vi "IO_Switch_#2(S2).vi"(8 "error in":errorcluster, 10 "Output":T1(ring)=enum."AVR (J3)", 11 "Input":T2(ring)=enum."Splitter") -> (0 "error out":errorcluster, 2 "Verfied":bool, 3 "Switches":string)   [LabVIEW 2012]
panel:
  # "IO Switch #2 (S2)"
  # "Switch Output"
  # "Switch Input"
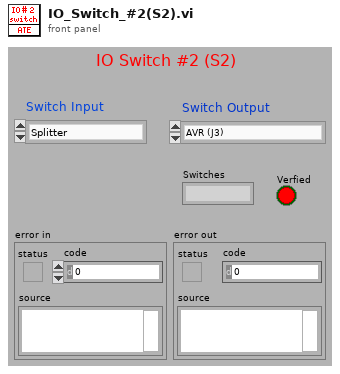
[diagram p1: front panel]
types:
  T1 = enum16{"NONE", "AVR (J3)", "Signal Out Switch (S3)", "Power Meter Switch (S5)", "Reversing Switch", "2W Term (TM1)"}
  T2 = enum16{"NONE", "AVR (J3)", "Splitter", "Signal Out Switch (S3)", " 2W Term (TM1)", "Reversing Switch", "Power Meter Switch"}
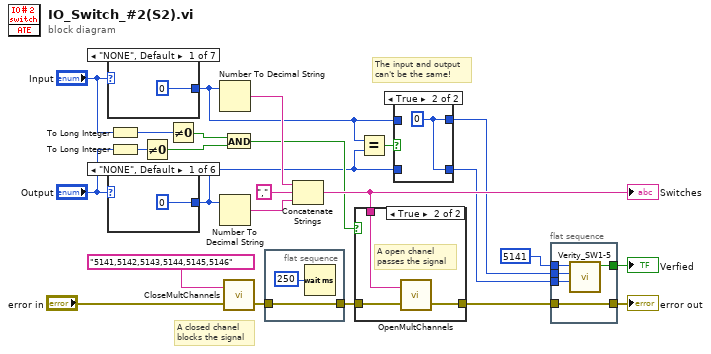
[diagram p0: block diagram]
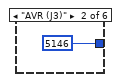
[diagram p3: hidden frame]
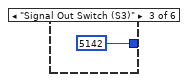
[diagram p4: hidden frame]
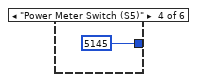
[diagram p5: hidden frame]
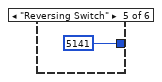
[diagram p6: hidden frame]
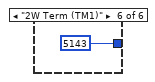
[diagram p7: hidden frame]
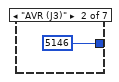
[diagram p8: hidden frame]
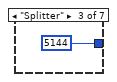
[diagram p9: hidden frame]
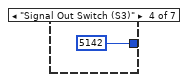
[diagram p10: hidden frame]
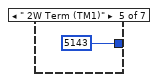
[diagram p11: hidden frame]
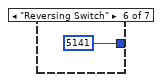
[diagram p12: hidden frame]
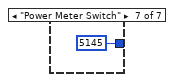
[diagram p13: hidden frame]
diagram:
  # "The input and output\ncan't be the same!"
  # "A closed chanel\nblocks the signal"
  n1 = case shown="\"NONE\", Default" "Input" {
    tunnel: [0 ("Switch ID") 5146 ("Switch ID") 5144 ("Switch ID") 5142 ("Switch ID") 5143 ("Switch ID") 5141 ("Switch ID") 5145 ("Switch ID")] -> w7
    frame "NONE", Default {
    }
    frame "AVR (J3)" {
    }
    frame "Splitter" {
    }
    frame "Signal Out Switch (S3)" {
    }
    frame " 2W Term (TM1)" {
    }
    frame "Reversing Switch" {
    }
    frame "Power Meter Switch" {
    }
  }
  n2 = case shown="\"NONE\", Default" "Output" {
    tunnel: [0 ("Switch ID") 5146 ("Switch ID") 5142 ("Switch ID") 5145 ("Switch ID") 5141 ("Switch ID") 5143 ("Switch ID")] -> w8
    frame "NONE", Default {
    }
    frame "AVR (J3)" {
    }
    frame "Signal Out Switch (S3)" {
    }
    frame "Power Meter Switch (S5)" {
    }
    frame "Reversing Switch" {
    }
    frame "2W Term (TM1)" {
    }
  }
  n3 = To Long Integer(number="Input") -> (32bit integer=w14:i32)
  n4 = To Long Integer(number="Output") -> (32bit integer=w13:i32)
  n5 = Not Equal To 0?(x=w13) -> (x != 0?=w12:bool)
  n6 = Not Equal To 0?(x=w14) -> (x != 0?=w11:bool)
  n7 = Number To Decimal String(number=w7) -> (decimal integer string=w17:string)  [unwired: 1 in]
  n8 = Number To Decimal String(number=w8) -> (decimal integer string=w18:string)  [unwired: 1 in]
  n9 = And(x=w11, y=w12) -> (x .and. y?=w10:bool)
  n10 = call "CloseMultChannels.vi"("error in (no error)"="error in", "Channels to be closed"="5141,5142,5143,5144,5145,5146" ("Channels to be opened")) -> ("error out"=w20:errorcluster)  [unwired: 1 in]
  n11 = flat-sequence {
    tunnel: w20 -> [w38]
    tunnel: [w38] -> w19
    frame #0 {
      n12 = Wait (ms)(milliseconds to wait=u32 250) -> ()  [unwired: 1 out]
    }
  }
  n13 = Concatenate Strings(w17, ",", w18) -> (w21:string)
  "Switches" <- w21
  n14 = case shown="True" w10 {
    tunnel: w19 -> [w40 w42]
    tunnel: w21 -> [_ w43]
    tunnel: [w40 w41] -> w2
    frame False {
    }
    frame True {
      # "A open chanel\npasses the signal"
      n15 = call "OpenMultChannels.vi"("error in (no error)"=w42, "Channels to be opened"=w43) -> ("error out"=w41:errorcluster)  [unwired: 1 in]
    }
  }
  n16 = Equal?(x=w7, y=w8) -> (x = y?=w9:bool)
  n17 = case shown="True" w9 {
    tunnel: w8 -> [w44 _]
    tunnel: [w44 w46] -> w4
    tunnel: w7 -> [w45 _]
    tunnel: [w45 w46] -> w3
    frame False {
    }
    frame True {
      w46 = 0 ("Switch ID")
    }
  }
  n18 = flat-sequence {
    tunnel: 5141 ("Switch ID") -> [w51]
    tunnel: w3 -> [w50]
    tunnel: w4 -> [w49]
    tunnel: [w48] -> w6
    tunnel: w2 -> [w47]
    tunnel: [w47] -> w1
    frame #0 {
      n19 = call "Verity_SW1-5.vi"("Output Switch ID"=w49, "Input Switch ID"=w50, "Base Switch ID"=w51) -> ("Verfied"=w48:bool)  [unwired: 7 in, 1 out]
    }
  }
  "error out" <- w1
  "Verfied" <- w6
